vi "Error Handler - Acquisition Message Loop.vi"(7 "Loop":string, 8 "error in (no error)":errorcluster, 9 "Ignore Errors (Runtime)":i32[](array[numeric]), 10 "Database":refnum<queue>, 11 "Message Queue":refnum<queue>) -> (0 "dup error in":errorcluster, 3 "dup Message Queue":refnum<queue>)   [LabVIEW 2026, in "Acquisition.lvlib"]
doc: "Process an error that occurred in the Acquisition Message Loop, either by ignoring it, or generating an \"Error\" message."
uses:
  Acquisition.lvlib
  support/Message Queue/Message Cluster.ctl
  support/Message Queue/Message Queue.lvlib
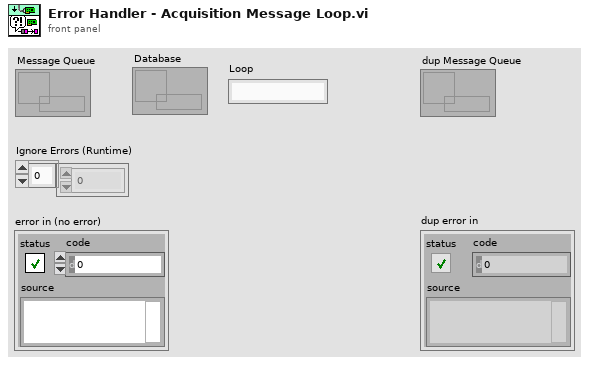
[diagram p1: front panel]
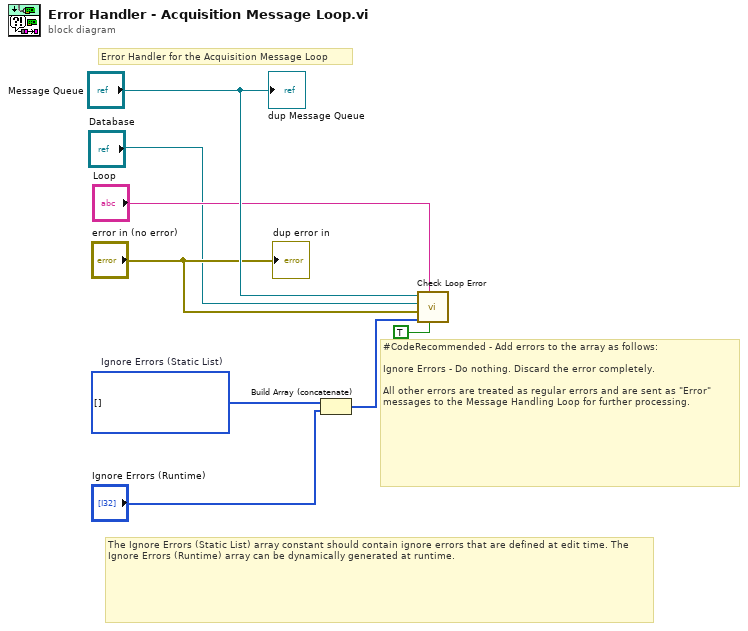
[diagram p0: block diagram]
diagram:
  w7 = i32[] []  # Ignore Errors (Static List)
  # "The Ignore Errors (Static List) array constant should contain ignore errors that are defined at edit time. The Ignore Errors (Runtime) array can be dynamically generated at runtime."
  # "#CodeRecommended - Add errors to the array as follows:\n\nIgnore Errors - Do nothing. Discard the error completely.\n\nAll other errors are treated as regular errors and are sent as \"Error\" messages to the Message Handling Loop for further processing."
  # "Error Handler for the Acquisition Message Loop"
  n1 = Build Array (concatenate)(w7, "Ignore Errors (Runtime)") -> (w5:i32[])
  n2 = call "Check Loop Error.vi"("Exit on Error? (F)"=TRUE, "Loop Name"="Loop", "Ignore Errors"=w5, "error to process"="error in (no error)", "Database"="Database", "Message Queue"="Message Queue") -> ()  [unwired: 4 in, 2 out]
  "dup Message Queue" <- "Message Queue"
  "dup error in" <- "error in (no error)"
